vi "Read CS++Factory.vi"(8 "Error In":errorcluster, 11 "CS++RTWatchdogActor in":refnum<class "CS++RTWatchdogActor.lvclass">) -> (0 "Error Out":errorcluster, 2 "CS++Factory":refnum<class "CS++Factory.lvclass">, 3 "CS++RTWatchdogActor out":refnum<class "CS++RTWatchdogActor.lvclass">)   [LabVIEW 2016, in "CS++RTWatchdog.lvlib" / "CS++RTWatchdogActor.lvclass"]
doc: "Read Factory from attribute."
uses:
  CS++RTWatchdogActor.lvclass
  CSPP_Core/Classes/CS++BaseClasses/Factory/CS++Factory.lvclass
  CS++RTWatchdogActor.lvclass/CS++RTWatchdogActor.ctl
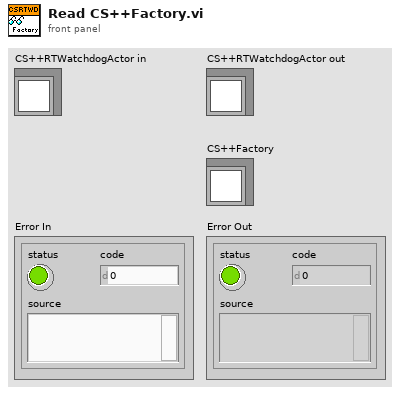
[diagram p1: front panel]
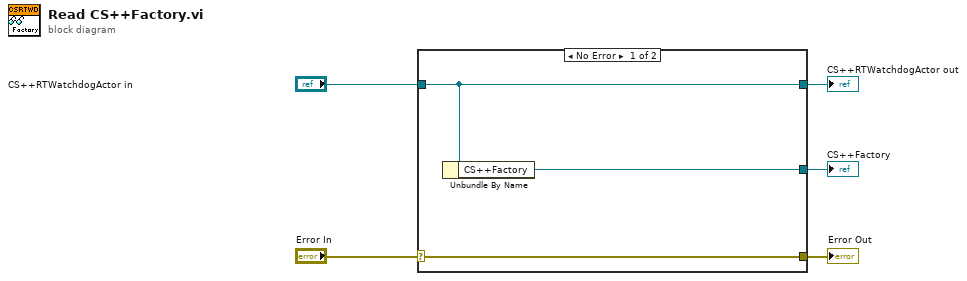
[diagram p0: block diagram]
diagram:
  n1 = case shown="No Error" "Error In" {
    selector: "Error In" -> [w8 w9]
    tunnel: [w8 w9] -> w4
    tunnel: [w7 w10] -> w2
    tunnel: "CS++RTWatchdogActor in" -> [w7 w10]
    tunnel: [w6 _] -> w1
    frame No Error {
      n2 = Unbundle By Name(w7) -> ("CS++Factory"=w6:refnum<class "CS++Factory.lvclass">)
    }
    frame Error {
    }
  }
  "Error Out" <- w4
  "CS++RTWatchdogActor out" <- w2
  "CS++Factory" <- w1
